vi "PickImage.vi"(1 "Get/Set":bool, 2 "Images (input)":T1 {"Coefficients (2D)" format="%.2f"}) -> (0 "Image (output)":T1 {"Coefficients (2D)" format="%.2f"})   [LabVIEW 2009]
uses:
  PickImage.ctl
  <vilib>/vision/Image Controls.llb/IMAQ Image.ctl
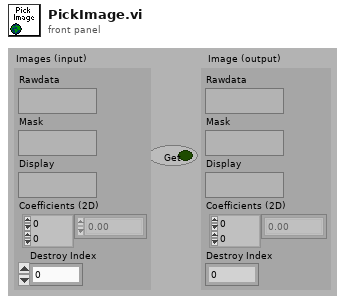
[diagram p1: front panel]
types:
  T1 = typedef "PickImage.ctl" = cluster{"Rawdata":T2, "Mask":T2, "Display":T2, "Coefficients (2D)":sgl[][], "Destroy Index":u32}
  T2 = typedef "IMAQ Image.ctl" = refnum<image>
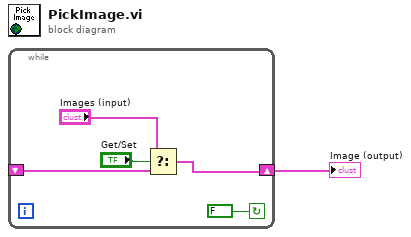
[diagram p0: block diagram]
diagram:
  n1 = while {
    shift-right: [w4] -> w1
    shift-left: _ -> [w5]
    stop <- FALSE continue-if-true
    n2 = Select(t="Images (input)", s="Get/Set", f=w5) -> (s? t:f=w4:T1)
  }
  "Image (output)" <- w1
